vi "GEvt-Generate Message Log.vi"(0 "CSM Global Log Event":T5, 1 "Current State":string, 2 "Arguments":string, 3 "Source Module":string, 5 "Type":T1, 6 "Name (\"\" to Use UUID)":string, 10 "CSM:LogFilter.lvclass":refnum<class "LogFilter.lvclass">) -> (14 "CSM Global Log Event Out":T5, 16 "Event Data":T2={"Name (\"\" to Use UUID)"="", "Current State"="", "Arguments"="", "Source Message"={"‘State"="", "’Arguments"="", "’Error"={"status"=FALSE, "code"=0, "source"=""}}, "Source Module"="", "Complete(T)/Start(F)"=FALSE, "LogType"=enum."State Change", "Time Stamp"=timestamp(0 s since 1904-01-01)})   [LabVIEW 2017, in "Communicable State Machine.lvlib"]
doc: "### GEvt-Generate Status Log.vi\n\n-- <b>Controls</b> --\n- <b>CSM Global Log Event</b>:\n- <b>Current State</b>:\n- <b>Arguments</b>:\n- <b>Name(\"\" to use uuid)</b>:\n- <b>CSM:LogFilter.lvclass</b>:\n\n-- <b>Indicators</b> --\n- <b>CSM Global Log Event out</b>:\n- <b>event data</b>:"
uses:
  Communicable State Machine.lvlib
  GEvt-Refs.ctl
  Typedef/_CSM_GlobalLog_MSG.ctl
  Typedef/_CSM_Response Source Message.ctl
  Typedef/_CSM_GlobalLog_MSG_TYPE.ctl
  LogFilter/LogFilter.lvclass
  AdvanceAPI/CSM - Message Type.ctl
  LogFilter/LogFilter - Check.vi
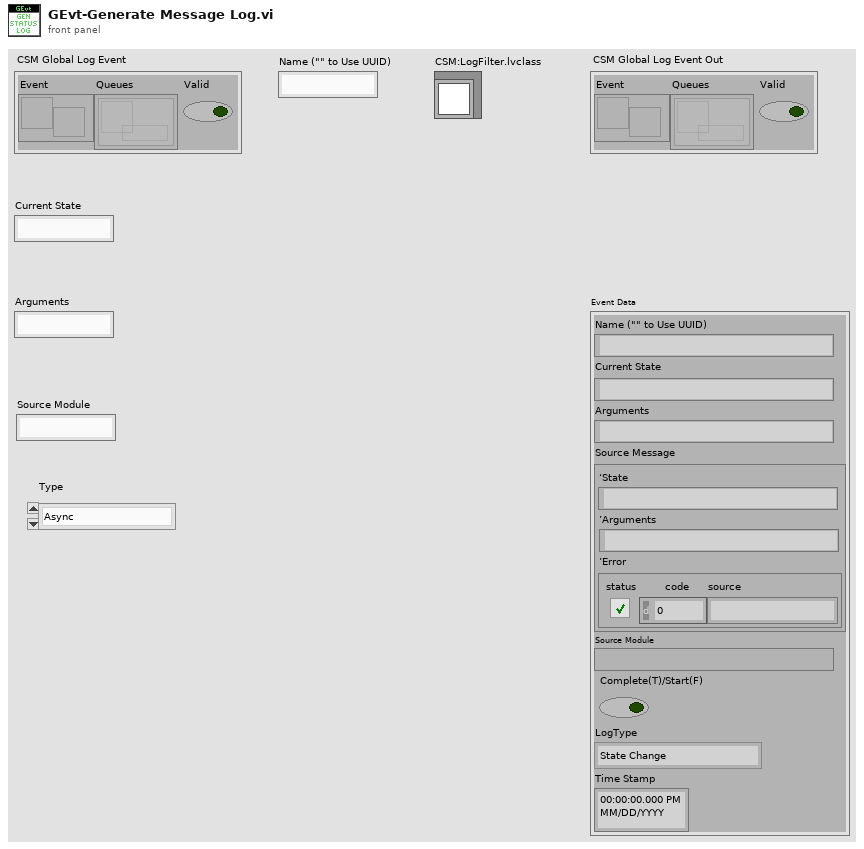
[diagram p1: front panel]
types:
  T1 = typedef "Communicable State Machine.lvlib/CSM - Message Type.ctl" = enum16{"Async", "Async without Reply", "Sync"}
  T2 = typedef "Communicable State Machine.lvlib/_CSM_GlobalLog_MSG.ctl" = cluster{"Name (\"\" to Use UUID)":string, "Current State":string, "Arguments":string, "Source Message":T3, "Source Module":string, "Complete(T)/Start(F)":bool, "LogType":T4, "Time Stamp":timestamp}
  T3 = typedef "Communicable State Machine.lvlib/_CSM_Response Source Message.ctl" = cluster{"‘State":string, "’Arguments":string, "’Error":errorcluster}
  T4 = typedef "Communicable State Machine.lvlib/_CSM_GlobalLog_MSG_TYPE.ctl" = enum16{"User Log", "State Change", "Status", "Interrupt", "Register", "Unregister", "Error Log", "Module Created", "Module Destroyed", "Async Message", "No-Rep Async Message", "Sync Message"}
  T5 = typedef "Communicable State Machine.lvlib/GEvt-Refs.ctl" = cluster{"Event":refnum<user-event>, "Queues":refnum<queue>[], "Valid":bool}
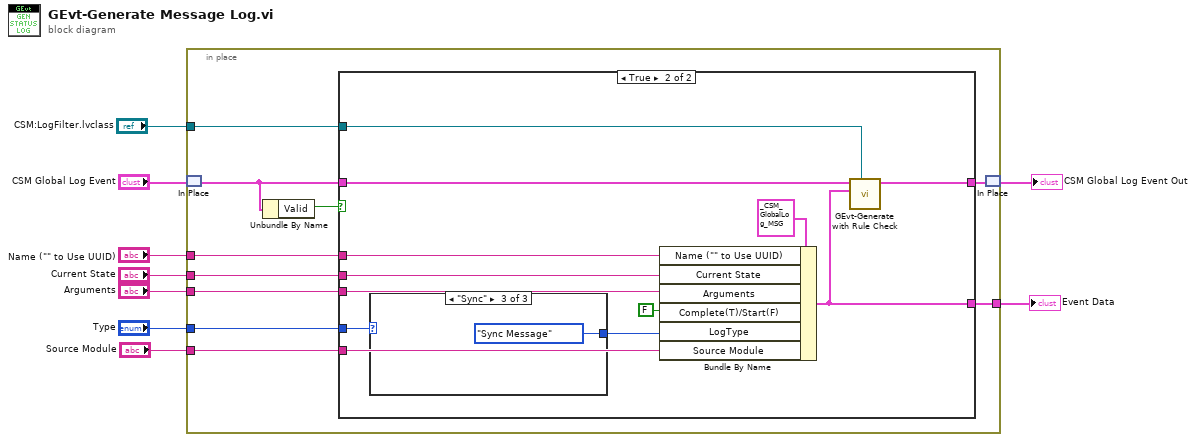
[diagram p0: block diagram]
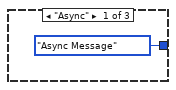
[diagram p3: hidden frame]
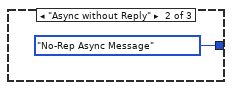
[diagram p4: hidden frame]
diagram:
  n1 = in-place {
    in-place-border: [w18] -> w7
    in-place-border: "Name (\"\" to Use UUID)" -> [w17]
    in-place-border: "Current State" -> [w16]
    in-place-border: "Arguments" -> [w15]
    in-place-border: "CSM:LogFilter.lvclass" -> [w14]
    in-place-border: "Source Module" -> [w11]
    in-place-border: "Type" -> [w10]
    n2 = in-place-match #1("CSM Global Log Event") -> (w13:T5)
    n3 = Unbundle By Name(w13) -> ("Valid"=w12:bool)
    n4 = case shown="True" w12 {
      tunnel: w13 -> [w20 w32]
      tunnel: [w20 w31] -> w19
      tunnel: [_ w24] -> w18
      tunnel: w17 -> [_ w28]
      tunnel: w16 -> [_ w27]
      tunnel: w15 -> [_ w26]
      tunnel: w14 -> [_ w25]
      tunnel: w11 -> [_ w23]
      tunnel: w10 -> [_ w22]
      frame False {
      }
      frame True {
        n5 = case shown="\"Sync\"" w22 {
          tunnel: [_CSM_GlobalLog_MSG_TYPE."Async Message" ("LogType") _CSM_GlobalLog_MSG_TYPE."No-Rep Async Message" ("LogType") _CSM_GlobalLog_MSG_TYPE."Sync Message" ("LogType")] -> w21
          frame "Async" {
          }
          frame "Async without Reply" {
          }
          frame "Sync" {
          }
        }
        n6 = Bundle By Name(cluster=T2 {"Name (\"\" to Use UUID)"="", "Current State"="", "Arguments"="", "Source Message"={"‘State"="", "’Arguments"="", "’Error"={"status"=FALSE, "code"=0, "source"=""}}, "Source Module"="", "Complete(T)/Start(F)"=FALSE, "LogType"=enum."State Change", "Time Stamp"=timestamp(0 s since 1904-01-01)} ("event data"), "Name (\"\" to Use UUID)"=w28, "Current State"=w27, "Arguments"=w26, "Complete(T)/Start(F)"=FALSE, "LogType"=w21, "Source Module"=w23) -> (w24:T2)
        n7 = call "GEvt-Generate with Rule Check.vi"("LogFilter In"=w25, "Event Data"=w24, "CSM Global Log Event In"=w32) -> ("CSM Global Log Event Out"=w31:T5)  [unwired: 8 in]
      }
    }
    n8 = in-place-match #1(w19) -> (→"CSM Global Log Event Out":T5)
  }
  "Event Data" <- w7
